vi "Modbus Multi-Read U8.vi"(7 "Slave Address":u8, 8 "error in (no error)":errorcluster, 9 "Number of U8 to read":i32 format="%x", 10 "Register Start Address":u16 format="%x", 11 "VISA resource in":refnum<visa-resource-name>) -> (0 "error out":errorcluster, 1 "Output data [U8]":u8[](array[numeric]), 3 "VISA resource out":refnum<visa-resource-name>)   [LabVIEW 2024, in "Voegtlin_NI_SMART_Modbus_Drivers.lvlib"]
doc: "Lese die geforderte Anzahl U8-Werte ab der angegebenen Startadresse des selektierten Geraetes aus.\nDer COM-Port muss dazu initialisiert sein (benutze\" Modbus Init.vi\")."
uses:
  Voegtlin_NI_SMART_Modbus_Drivers.lvlib
  Enums/Modbus Comm.ctl
panel:
  out "Read register data\n U16 (array)":u16[](array[numeric])
  # "Internal Data"
  # "Output Data"
  # "Input Data"
  # "(Inputmaske in HEX)"
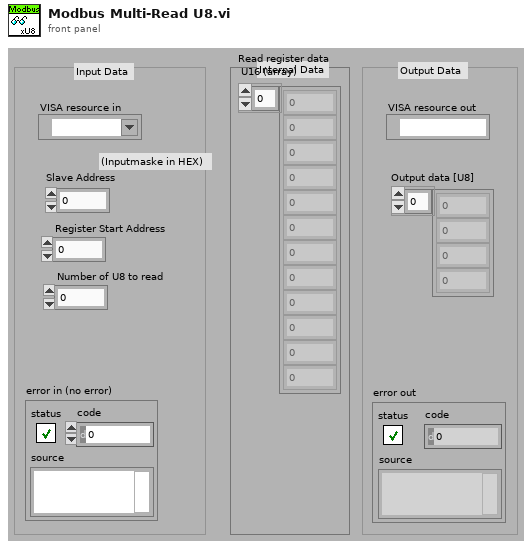
[diagram p1: front panel]
types:
  T1 = typedef "Voegtlin_NI_SMART_Modbus_Drivers.lvlib/Modbus Comm.ctl" = enum16{"Init", "Read", "Write", "Exit"}
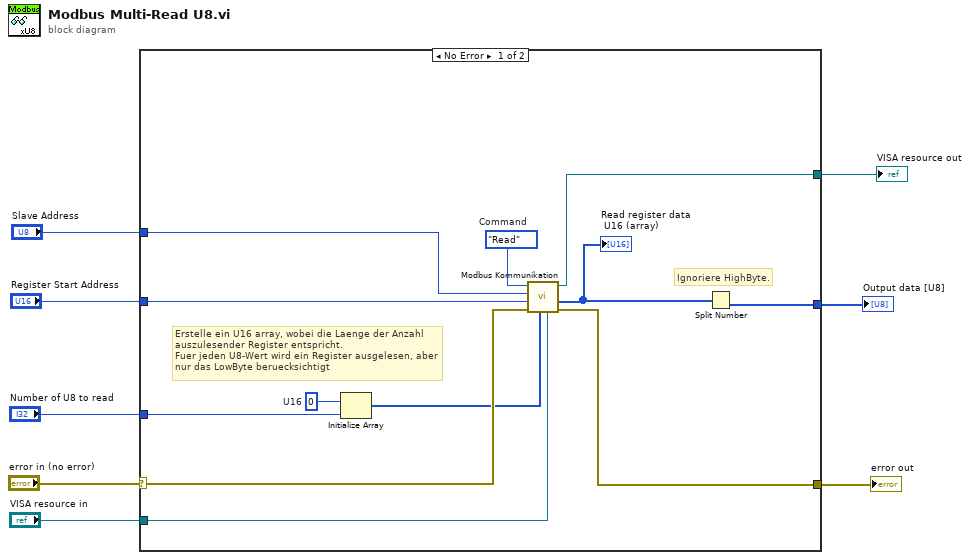
[diagram p0: block diagram]
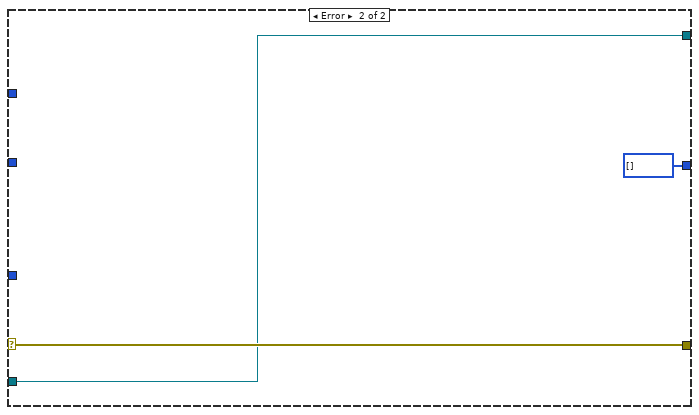
[diagram p2: hidden frame]
diagram:
  n1 = case shown="No Error" "error in (no error)" {
    selector: "error in (no error)" -> [w14 w23]
    tunnel: "Register Start Address" -> [w12 _]
    tunnel: [w20 w23] -> w7
    tunnel: [w16 u8[] []] -> w6
    tunnel: "Number of U8 to read" -> [w15 _]
    tunnel: "Slave Address" -> [w11 _]
    tunnel: "VISA resource in" -> [w10 w21]
    tunnel: [w9 w21] -> w1
    frame No Error {
      w18 = u16 0  # U16
      w19 = Modbus_Comm."Read"  # Command
      # "Ignoriere HighByte."
      # "Erstelle ein U16 array, wobei die Laenge der Anzahl auszulesender Register entspricht.\nFuer jeden U8-Wert wird ein Register ausgelesen, aber nur das LowByte beruecksichtigt"
      n2 = Initialize Array(w18, w15) -> (w13:u16[])
      n3 = call "Modbus Kommunikation.vi"("VISA resource in"=w10, "Data In / #Reads [U16]"=w13, "error in (no error)"=w14, "Register Start Address"=w12, "Slave Address"=w11, "Command"=w19) -> ("error out"=w20:errorcluster, "Data Out [U16]"=w17:u16[], "VISA resource out"=w9:refnum<visa-resource-name>)  [unwired: 3 in]
      "Read register data\n U16 (array)" <- w17
      n4 = Split Number(x=w17) -> (lo(x)=w16:u8[])  [unwired: 1 out]
    }
    frame Error {
    }
  }
  "error out" <- w7
  "Output data [U8]" <- w6
  "VISA resource out" <- w1
